vi "Stage 4.2 Adding common data init and  startstop on aqn.vi"() -> ()   [LabVIEW 2020]
panel:
  out "Process Error":errorcluster
  out "error out":errorcluster
  out "error out Hardware":errorcluster
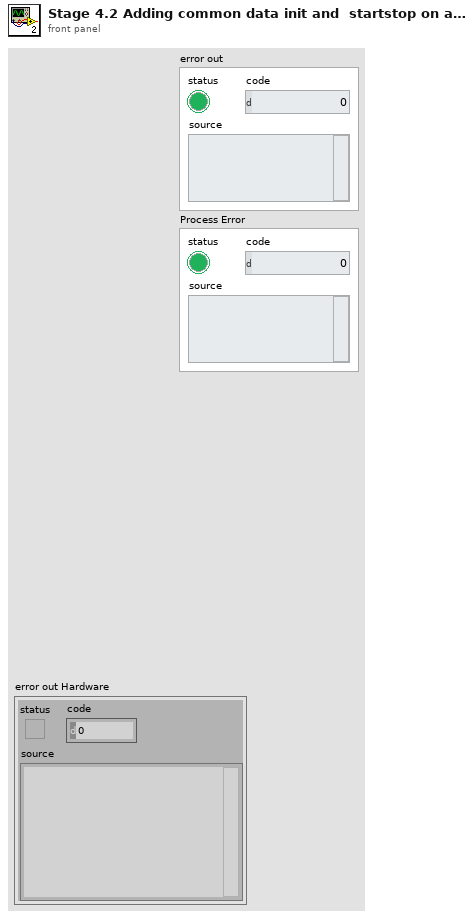
[diagram p1: front panel]
types:
  T1 = typedef "HRM-Stage4-init_cluster.ctl" = cluster{"config":T2, "User Events":T3}
  T2 = typedef "HRM-stage4-config_data.ctl" = cluster{"Run AQN?":bool}
  T3 = typedef "HRM-Stage4-User_events.ctl" = cluster{"Signal to remove":refnum<user-event>, "Sample size":refnum<user-event>, "Filtered wf":refnum<user-event>, "Unfiltered wf":refnum<user-event>, "Raw wf":refnum<user-event>, "Pulse":refnum<user-event>, "Stop":refnum<user-event>, "Feedback":refnum<user-event>, "Run Aqn?":refnum<user-event>, "Clear":refnum<user-event>, "Peak Det. Set.":refnum<user-event>}
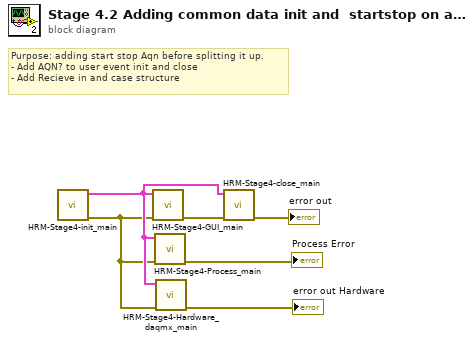
[diagram p0: block diagram]
diagram:
  # "Purpose: adding start stop Aqn before splitting it up.\n- Add AQN? to user event init and close\n- Add Recieve in and case structure"
  n1 = call "HRM-Stage4-init_main.vi"() -> ("error out"=w1:errorcluster, "Init cluster"=w2:T1)  [unwired: 10 in]
  n2 = call "HRM-Stage4-GUI_main.vi"("error in (no error)"=w1, "Init cluster"=w2) -> ("error out"=w3:errorcluster)  [unwired: 9 in]
  n3 = call "HRM-Stage4-Process_main.vi"("error in (no error)"=w1, "Init cluster"=w2) -> ("error out"=→"Process Error":errorcluster)  [unwired: 9 in]
  n4 = call "HRM-Stage4-Hardware_daqmx_main.vi"("error in (no error)"=w1, "Init cluster"=w2) -> ("error out"=→"error out Hardware":errorcluster)  [unwired: 9 in]
  n5 = call "HRM-Stage4-close_main.vi"("error in (no error)"=w3, "Init cluster"=w2) -> ("error out"=→"error out":errorcluster)  [unwired: 9 in]
